vi "ArmControl.vi"(8 "Last Increment time":dbl, 9 "Current time":dbl, 10 "Joystick":dbl, 11 "Increment":dbl) -> (0 "Last Time":u32, 3 "Increment Amount":dbl)   [LabVIEW 2015]
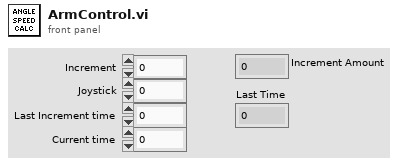
[diagram p1: front panel]
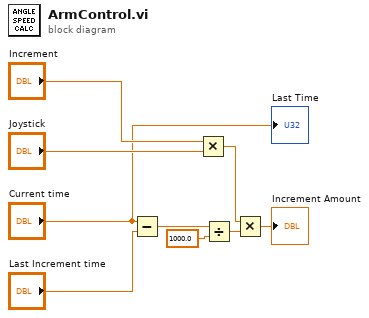
[diagram p0: block diagram]
diagram:
  n1 = Subtract(x="Current time", y="Last Increment time") -> (x-y=w8:dbl)
  n2 = Multiply(x="Increment", y="Joystick") -> (x*y=w4:dbl)
  n3 = Divide(x=w8, y=1000.0) -> (x/y=w2:dbl)
  n4 = Multiply(x=w4, y=w2) -> (x*y=→"Increment Amount":dbl)
  "Last Time" <- "Current time"
